vi "Retrieve RTV [by name].vi"(0 "RTV name":string, 11 "error in (no error)":errorcluster) -> (4 "Data":variant, 6 "Scope":i64, 8 "RTV present?":bool, 15 "error out":errorcluster)   [LabVIEW 2016, in "RT Variables.lvclass"]
uses:
  RT Variables.lvclass
  protected/Singleton Action.ctl
  RT Variables.lvclass/RT Variables.ctl
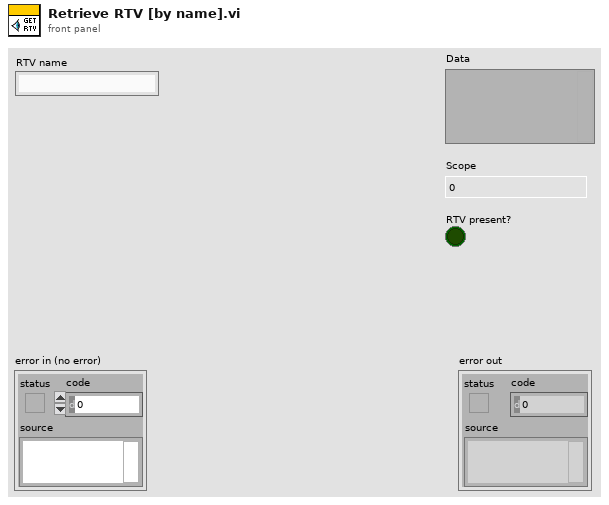
[diagram p1: front panel]
types:
  T1 = typedef "RT Variables.lvclass/Singleton Action.ctl" = enum16{"Get", "Set"}
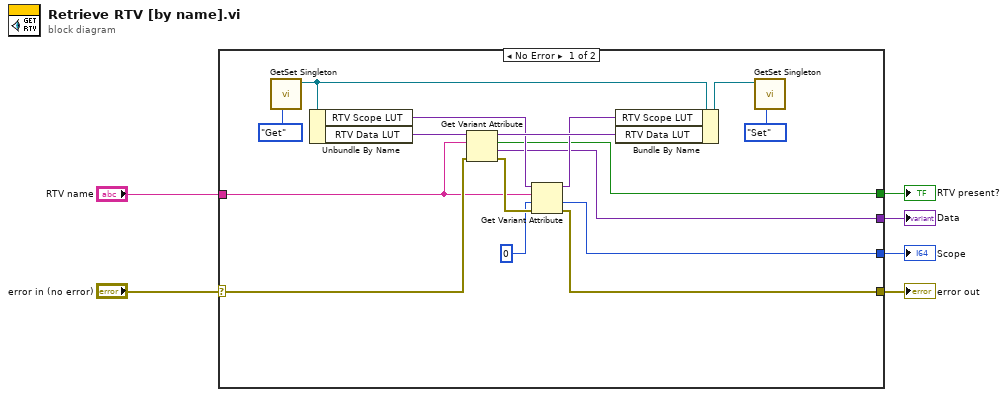
[diagram p0: block diagram]
diagram:
  n1 = case shown="No Error" "error in (no error)" {
    selector: "error in (no error)" -> [w16 w23]
    tunnel: [w12 w23] -> w5
    tunnel: "RTV name" -> [w11 _]
    tunnel: [w9 _] -> w3
    tunnel: [w8 _] -> w2
    tunnel: [w7 _] -> w1
    frame No Error {
      n2 = call "GetSet Singleton.vi"("Action"=Singleton_Action."Get") -> ("RT Variables out"=w20:refnum<class "RT Variables.lvclass">)  [unwired: 9 in, 1 out]
      n3 = Unbundle By Name(w20) -> ("RTV Scope LUT"=w15:variant, "RTV Data LUT"=w18:variant)
      n4 = Get Variant Attribute(Variant=w18, name=w11, error in=w16) -> (duplicate Variant=w17:variant, found=w7:bool, value=w8:variant, error out=w13:errorcluster)  [unwired: 1 in]
      n5 = Get Variant Attribute(Variant=w15, name=w11, default value (empty Variant)=i64 0 ("Scope"), error in=w13) -> (duplicate Variant=w14:variant, value=w9:i64, error out=w12:errorcluster)  [unwired: 1 out]
      n6 = Bundle By Name(cluster=w20, "RTV Scope LUT"=w14, "RTV Data LUT"=w17) -> (w19:refnum<class "RT Variables.lvclass">)
      n7 = call "GetSet Singleton.vi"("Action"=Singleton_Action."Set", "RT Variables in"=w19) -> ()  [unwired: 8 in, 2 out]
    }
    frame Error {
    }
  }
  "error out" <- w5
  "Data" <- w2
  "Scope" <- w3
  "RTV present?" <- w1
